vi "Vector2DNormalize.vi"(10 "Vector":T1) -> (2 "Normalized Vector":T1)   [LabVIEW 2018]
uses:
  Vector2D.ctl
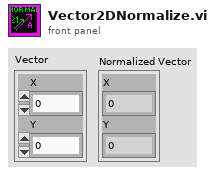
[diagram p1: front panel]
types:
  T1 = typedef "Vector2D.ctl" = cluster{"X":dbl, "Y":dbl}
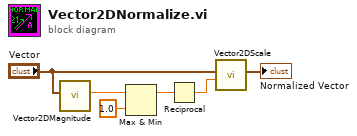
[diagram p0: block diagram]
diagram:
  n1 = call "Vector2DMagnitude.vi"("Vector"="Vector") -> ("Magnitude"=w2:dbl)  [unwired: 10 in]
  n2 = Max & Min(x=w2, y=1.0) -> (max(x,y)=w4:dbl)  [unwired: 1 out]
  n3 = Reciprocal(x=w4) -> (1/x=w1:dbl)
  n4 = call "Vector2DScale.vi"("Scale Factor"=w1, "Vector"="Vector") -> ("Scaled Vector"=→"Normalized Vector":T1)  [unwired: 9 in]
